vi "Compass.vi"(2 "theta (deg)":dbl(slide)=1.021405182655144e-14 scale=-180.0..180.0) -> (0 "new picture":picture)   [LabVIEW 2012]
uses:
  <vilib>/picture/picture.llb/Draw True-Color Pixmap.vi
panel:
  out "Picture":picture
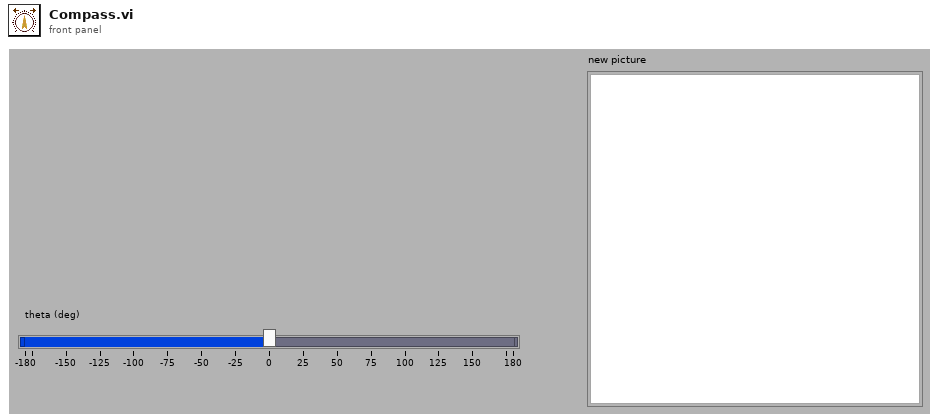
[diagram p1: front panel]
types:
  T1 = typedef "imagedata.ctl" = cluster{"image type":i32, "image depth":i32, "image":u8[], "mask":u8[], "colors":u32[], "Rectangle":cluster{"left":i16, "top":i16, "right":i16, "bottom":i16}}
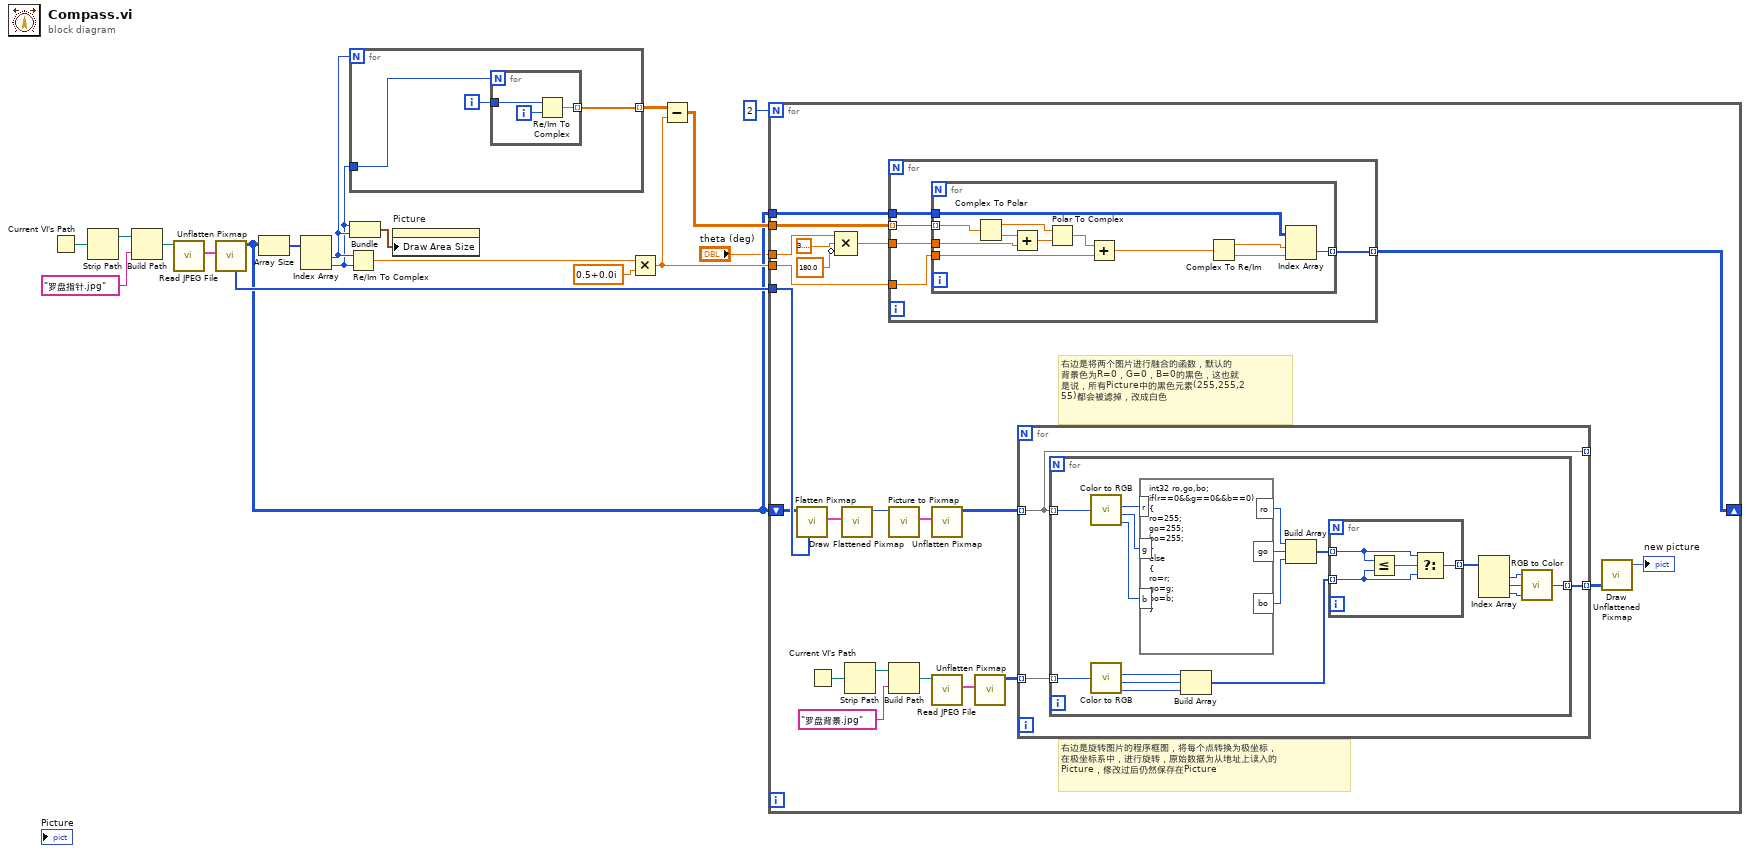
[diagram p0: block diagram]
diagram:
  n1 = Current VI's Path() -> (path=w6:path)
  n2 = Strip Path(path=w6) -> (stripped path=w5:path)  [unwired: 1 out]
  n3 = Build Path(base path=w5, name or relative path="罗盘指针.jpg" ("名称或相对路径")) -> (appended path=w3:path)
  n4 = call <vilib>:"Read JPEG File.vi"("path to JPEG file"=w3) -> ("image data"=w7:T1)  [unwired: 8 in, 2 out]
  n5 = call <vilib>:"Unflatten Pixmap.vi"("image data"=w7) -> ("24-bit pixmap"=w10:u32[][], "colors"=w11:u32[])  [unwired: 4 in, 5 out]
  n6 = Array Size(array=w10) -> (size(s)=w15:i32[])
  n7 = Index Array(array=w15) -> (element #1=w14:i32, element #2=w8:i32)  [unwired: 2 in]
  n8 = Re/Im To Complex(1:w8, 2:w14) -> (0:w16:cdb)
  n9 = for {
    N: w14 -> [_]
    tunnel: w8 -> [w21]
    tunnel: [w19] -> w18 mode=indexing
    i -> [w20]
    n10 = for {
      N: w21 -> [_]
      tunnel: w20 -> [w23]
      tunnel: [w22] -> w19 mode=indexing
      i -> [w24]
      n11 = Re/Im To Complex(1:w24, 2:w23) -> (0:w22:cdb)
    }
  }
  n12 = Bundle(w8, w14) -> (w9:cluster{i32, i32})  [unwired: 1 in]
  n13 = property on="Picture" class="Pict"("Draw Area Size"=w9) -> ()  [unwired: 2 in, 2 out]
  n14 = Multiply(x=w16, y=cdb 0.5+0.0i) -> (x*y=w13:cdb)
  n15 = Subtract(x=w18, y=w13) -> (x-y=w17:cdb[][])
  n16 = for {
    N: 2 -> [_]
    tunnel: w17 -> [w46]
    tunnel: w13 -> [w45]
    shift-right: [w43] -> _
    shift-left: w10 -> [w40]
    tunnel: w11 -> [w42]
    tunnel: w10 -> [w41]
    tunnel: "theta (deg)" -> [w25]
    # "右边是旋转图片的程序框图，将每个点转换为极坐标，\n在极坐标系中，进行旋转，原始数据为从地址上读入的\nPicture，修改过后仍然保存在Picture"
    # "右边是将两个图片进行融合的函数，默认的\n背景色为R=0，G=0，B=0的黑色，这也就\n是说，所有Picture中的黑色元素(255,255,2\n55)都会被滤掉，改成白色"
    n17 = call <vilib>:"Flatten Pixmap.vi"("colors"=w42, "24-bit pixmap"=w40) -> ("image data"=w44:T1)  [unwired: 9 in]
    n18 = Current VI's Path() -> (path=w34:path)
    n19 = Compound Arithmetic op=MULTIPLY(w25, 3.141592653589793, invert 180.0 ("value")) -> (w28:dbl)
    n20 = call <vilib>:"Draw Flattened Pixmap.vi"("image data"=w44) -> ("new picture"=w27:picture)  [unwired: 8 in]
    n21 = Strip Path(path=w34) -> (stripped path=w33:path)  [unwired: 1 out]
    n22 = for {
      tunnel: w28 -> [w51]
      tunnel: w41 -> [w50]
      tunnel: w45 -> [w49]
      tunnel: w46 -> [w48] mode=indexing
      tunnel: [w47] -> w43 mode=indexing
      n23 = for {
        tunnel: w50 -> [w57]
        tunnel: w51 -> [w60]
        tunnel: w49 -> [w54]
        tunnel: w48 -> [w53] mode=indexing
        tunnel: [w52] -> w47 mode=indexing
        n24 = Complex To Polar(r * e^(i*theta)=w53) -> (r=w63:dbl, theta=w62:dbl)
        n25 = Add(x=w62, y=w60) -> (x+y=w61:dbl)
        n26 = Polar To Complex(1:w61, 2:w63) -> (0:w59:cdb)
        n27 = Add(x=w59, y=w54) -> (x+y=w55:cdb)
        n28 = Complex To Re/Im(x + iy=w55) -> (x=w58:dbl, y=w56:dbl)
        n29 = Index Array(array=w57, index (row)=w58, index (col)=w56) -> (element=w52:u32)
      }
    }
    n30 = call <vilib>:"Picture to Pixmap.vi"("picture"=w27) -> ("image data"=w35:T1)  [unwired: 9 in, 1 out]
    n31 = Build Path(base path=w33, name or relative path="罗盘背景.jpg" ("名称或相对路径")) -> (appended path=w31:path)
    n32 = call <vilib>:"Unflatten Pixmap.vi"("image data"=w35) -> ("24-bit pixmap"=w26:u32[][])  [unwired: 4 in, 6 out]
    n33 = call <vilib>:"Read JPEG File.vi"("path to JPEG file"=w31) -> ("image data"=w39:T1)  [unwired: 8 in, 2 out]
    n34 = call <vilib>:"Unflatten Pixmap.vi"("image data"=w39) -> ("24-bit pixmap"=w36:u32[][])  [unwired: 4 in, 6 out]
    n35 = for {
      tunnel: [w64] -> _ mode=indexing
      tunnel: w36 -> [w66] mode=indexing
      tunnel: [w65] -> w38 mode=indexing
      tunnel: w26 -> [w64] mode=indexing
      n36 = for {
        tunnel: w64 -> [w78] mode=indexing
        tunnel: w66 -> [w77] mode=indexing
        tunnel: [w76] -> w65 mode=indexing
        n37 = call <vilib>:"Color to RGB.vi"("Color"=w78) -> ("R"=w72:u8, "G"=w71:u8, "B"=w70:u8)  [unwired: 1 out]
        n38 = call <vilib>:"Color to RGB.vi"("Color"=w77) -> ("R"=w84:u8, "G"=w83:u8, "B"=w82:u8)  [unwired: 1 out]
        n39 = formula code="int32 ro,go,bo;\nif(r==0&&g==0&&b==0)\n{\nro=255;\ngo=255;\nbo=255;\n}\nelse\n{\nro=r;\ngo=g;\nbo=b;\n}"("r"=w72, "g"=w71, "b"=w70) -> ("ro"=w69:i32, "go"=w68:i32, "bo"=w67:i32)
        n40 = Build Array(w84, w83, w82) -> (w74:u8[])
        n41 = Build Array(w69, w68, w67) -> (w75:i32[])
        n42 = for {
          tunnel: [w85] -> w73 mode=indexing
          tunnel: w75 -> [w87] mode=indexing
          tunnel: w74 -> [w86] mode=indexing
          n43 = Less Or Equal?(x=w87, y=w86) -> (x <= y?=w88:bool)
          n44 = Select(t=w87, s=w88, f=w86) -> (s? t:f=w85:i32)
        }
        n45 = Index Array(array=w73) -> (element #1=w81:i32, element #2=w80:i32, element #3=w79:i32)  [unwired: 3 in]
        n46 = call <vilib>:"RGB to Color.vi"("B"=w79, "G"=w80, "R"=w81) -> ("Color"=w76:u32)
      }
    }
    n47 = call-poly <vilib>:"Draw Unflattened Pixmap.vi"("data (RGB format)"=w38) -> ("new picture"=→"new picture":picture)  [unwired: 8 in]
  }
